vi "TCP READ DBL.vi"(8 "error In":errorcluster, 9 "Length":i32=100, 10 "Start Address":i32=1350, 11 "connection ID IN":refnum<k5>) -> (0 "error out":errorcluster, 2 "Data":dbl[](array[numeric]) format="%#.6f", 3 "connection ID OUT":refnum<k5>)   [LabVIEW 2015]
panel:
  out "concatenated string":string
  out "substring 3":string
  out "substring 2":string
  out "bytes written1":i32
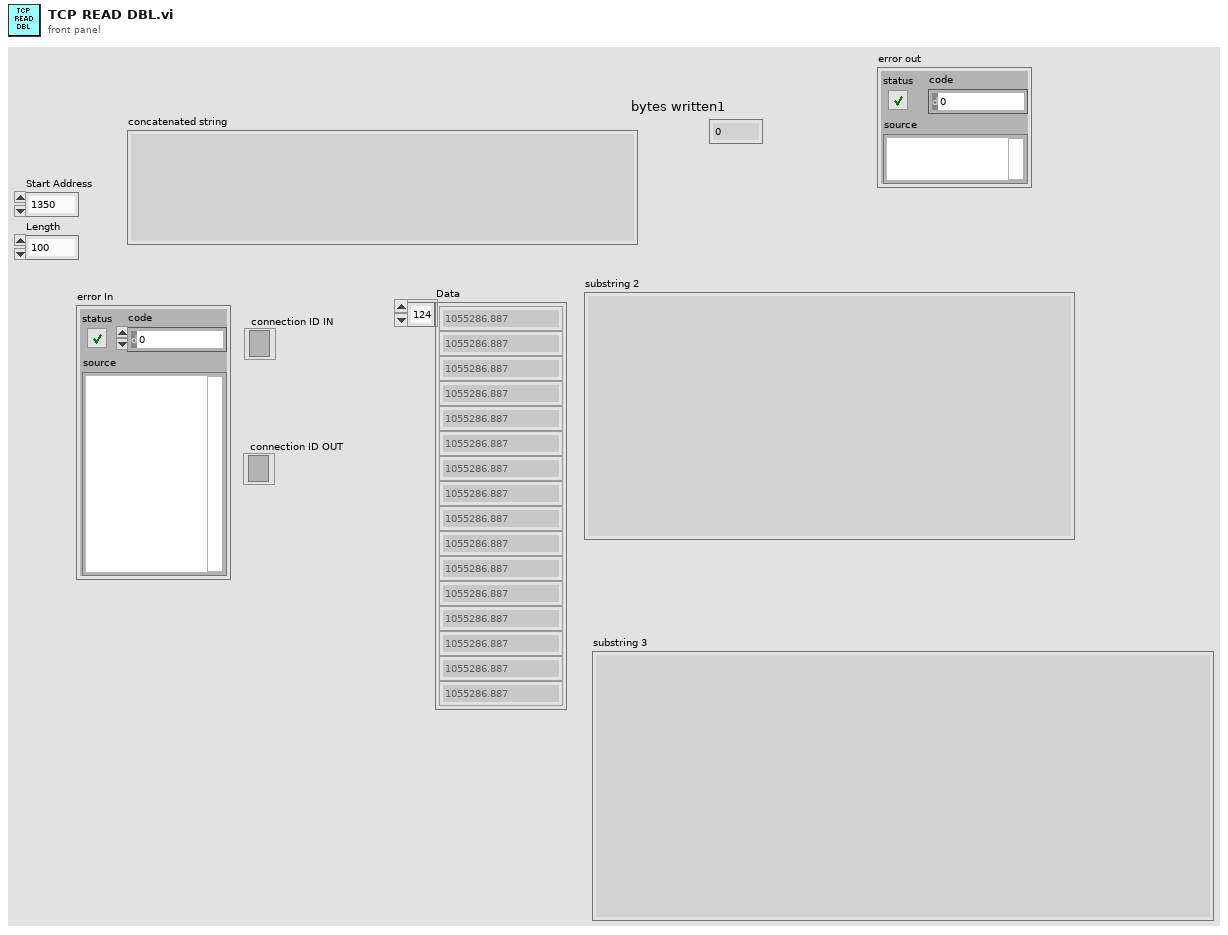
[diagram p1: front panel]
types:
  T1 = enum16{"Standard", "Buffered", "CRLF", "Immediate"}
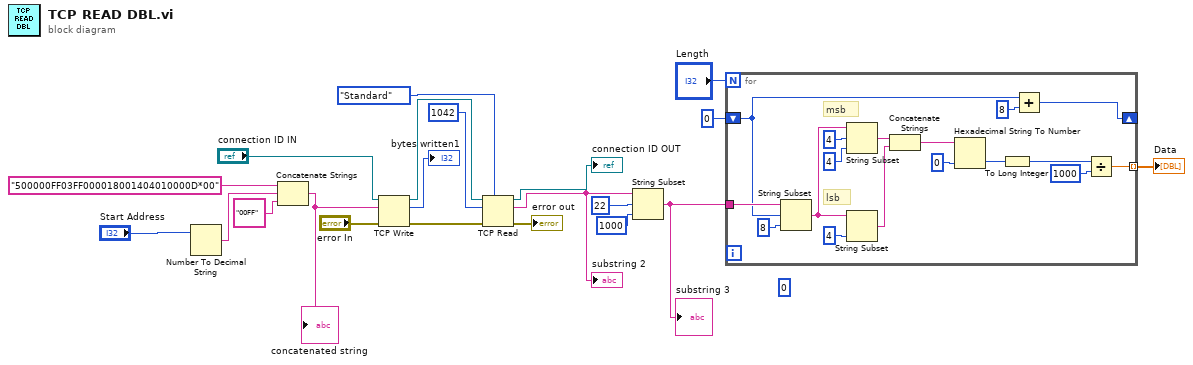
[diagram p0: block diagram]
diagram:
  (unwired) 0
  n1 = Number To Decimal String(number="Start Address") -> (decimal integer string=w18:string)  [unwired: 1 in]
  n2 = Concatenate Strings("500000FF03FF000018001404010000D*00", w18, "00FF" ("String")) -> (w20:string)
  "concatenated string" <- w20
  n3 = TCP Write(connection ID="connection ID IN", data in=w20, error in (no error)="error In") -> (connection ID out=w13:refnum<k5>, bytes written=→"bytes written1":i32, error out=w11:errorcluster)  [unwired: 1 in]
  n4 = TCP Read(connection ID=w13, bytes to read=1042, error in (no error)=w11, 7:T1."Standard" ("mode (standard)")) -> (connection ID out=→"connection ID OUT":refnum<k5>, data out=w9:string, error out=→"error out":errorcluster)  [unwired: 1 in]
  "substring 2" <- w9
  n5 = String Subset(string=w9, offset (0)=22, length (rest)=1000 ("length (rest)")) -> (substring=w1:string)
  "substring 3" <- w1
  n6 = for {
    N: "Length" -> [_]
    shift-right: [w38] -> _
    shift-left: 0 -> [w35]
    tunnel: w1 -> [w36]
    tunnel: [w22] -> w2 mode=indexing
    # "lsb"
    # "msb"
    n7 = String Subset(string=w36, offset (0)=w35, length (rest)=8 ("length (rest)")) -> (substring=w30:string)
    n8 = String Subset(string=w30, offset (0)=4, length (rest)=4 ("length (rest)")) -> (substring=w29:string)
    n9 = String Subset(string=w30, length (rest)=4 ("length (rest)")) -> (substring=w28:string)  [unwired: 1 in]
    n10 = Concatenate Strings(w29, w28) -> (w27:string)
    n11 = Hexadecimal String To Number(string=w27, default (0uL)=u32 0 ("default (0 U32)")) -> (number=w23:u32)  [unwired: 1 in, 1 out]
    n12 = To Long Integer(number=w23) -> (32bit integer=w24:i32)
    n13 = Add(x=w35, y=8) -> (x+y=w38:i32)
    n14 = Divide(x=w24, y=u32 1000) -> (x/y=w22:dbl)
  }
  "Data" <- w2
